vi "PH_PILS.get Status of GUI referenced Boolean Tags.vi"(2 "Tags":cluster{"GUI Ref":refnum<vi>, "Status":i32}[](array[cluster]), 3 "Tagname":string, 5 "error in":errorcluster) -> (16 "GUI Ref":refnum<vi>, 17 "Status":i32, 18 "index of element":i32, 19 "error out":errorcluster)   [LabVIEW 2014, in "PH_PILS.lvlib"]
doc: "This VI gets status, array position and GUI ref of the referenced tagname out of the array where the name is set to be the GUI ref."
uses:
  PH_PILS.lvlib
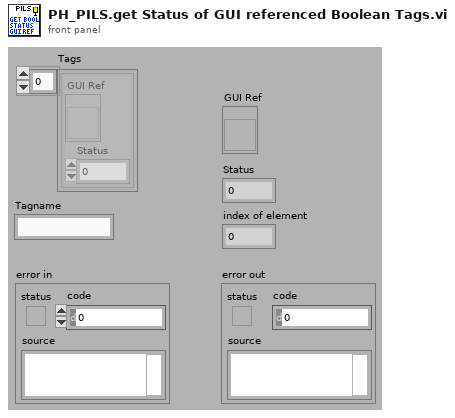
[diagram p1: front panel]
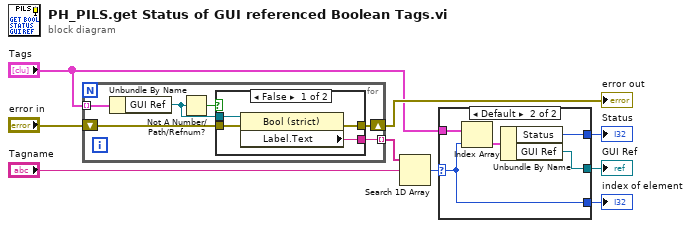
[diagram p0: block diagram]
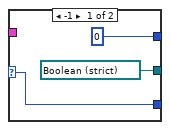
[diagram p2: hidden frame]
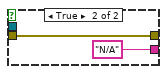
[diagram p3: hidden frame]
diagram:
  n1 = for {
    tunnel: "Tags" -> [w15] mode=indexing
    shift-right: [w11] -> w7
    shift-left: "error in" -> [w14]
    tunnel: [w10] -> w1 mode=indexing
    n2 = Unbundle By Name(w15) -> ("GUI Ref"=w12:refnum<vi>)
    n3 = Not A Number/Path/Refnum?(number/path/refnum=w12) -> (NaN/Path/Refnum?=w13:bool)
    n4 = case shown="False" w13 {
      tunnel: w12 -> [w19 _]
      tunnel: w14 -> [w18 w21]
      tunnel: [w17 w21] -> w11
      tunnel: [w16 "N/A" ("Label.Text")] -> w10
      frame False {
        n5 = property class="Bool (strict)"(reference=w19, error in=w18) -> (error out=w17:errorcluster, "Label.Text"=w16:string)  [unwired: 1 out]
      }
      frame True {
      }
    }
  }
  "error out" <- w7
  n6 = Search 1D Array(1D array=w1, element="Tagname") -> (index of element=w3:i32)  [unwired: 1 in]
  n7 = case shown="Default" w3 {
    selector: w3 -> [w24 w25]
    tunnel: "Tags" -> [_ w29]
    tunnel: [0 ("Status") w27] -> w9
    tunnel: [refnum<vi> refnum ("GUI Ref") w26] -> w5
    tunnel: [w24 w25] -> w2
    frame -1 {
    }
    frame Default {
      n8 = Index Array(array=w29, index=w25) -> (element=w28:cluster{"GUI Ref":refnum<vi>, "Status":i32})
      n9 = Unbundle By Name(w28) -> ("Status"=w27:i32, "GUI Ref"=w26:refnum<vi>)
    }
  }
  "Status" <- w9
  "index of element" <- w2
  "GUI Ref" <- w5
